vi "Grafica- Sin.vi"() -> ()   [LabVIEW 2020]
panel:
  out "Waveform Chart":dbl(graph)
  in  "stop":bool
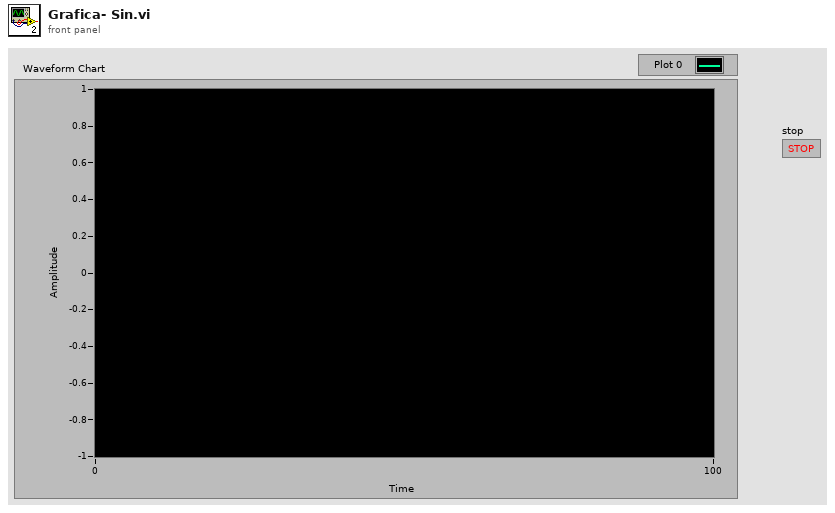
[diagram p1: front panel]
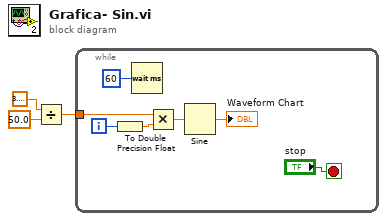
[diagram p0: block diagram]
diagram:
  n1 = Divide(x=3.141592653589793, y=50.0 ("x/y")) -> (x/y=w1:dbl)
  n2 = while {
    tunnel: w1 -> [w8]
    i -> [w10]
    stop <- "stop" stop-if-true
    n3 = To Double Precision Float(number=w10) -> (double precision float=w9:dbl)
    n4 = Wait (ms)(milliseconds to wait=u32 60 ("millisecond timer value")) -> ()  [unwired: 1 out]
    n5 = Multiply(x=w8, y=w9) -> (x*y=w5:dbl)
    n6 = Sine(x=w5) -> (sin(x)=→"Waveform Chart":dbl)
  }
